vi "Reevaluate Target.vi"(4 "Delay Time (s)":dbl=1.0, 11 "error in (no error)":errorcluster) -> (2 "What to do":string, 3 "error out (no error)":errorcluster)   [LabVIEW 2015]
uses:
  Robot Global Data.vi
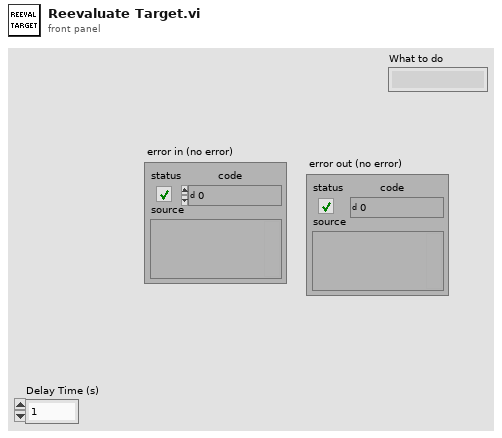
[diagram p1: front panel]
types:
  T1 = cluster{"Goal Left":dbl, "Goal Right":dbl, "Goal Width":dbl}
  T2 = typedef "Relevant Data.ctl" = cluster{"Area":dbl, "CH Area":dbl, "BR Width":dbl, "BR Height":dbl, "BR Left":dbl, "BR Right":dbl}
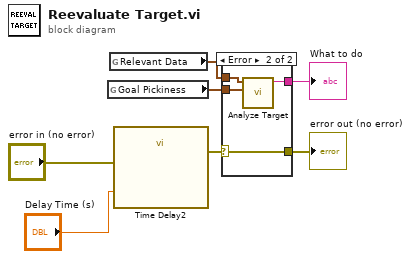
[diagram p0: block diagram]
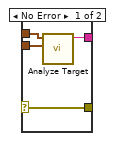
[diagram p2: hidden frame]
diagram:
  n1 = global read "Robot Global Data.vi" "Goal Pickiness"() -> (w3:T1)
  n2 = global read "Robot Global Data.vi" "Relevant Data"() -> (w4:T2[])
  n3 = call "Time Delay2"("error in (no error)"="error in (no error)", "Delay Time (s)"="Delay Time (s)") -> ("error out"=w5:errorcluster)  [unwired: 9 in]
  n4 = case shown="Error" w5 {
    selector: w5 -> [w8 w12]
    tunnel: w4 -> [w11 w15]
    tunnel: w3 -> [w10 w14]
    tunnel: [w9 w13] -> w2
    tunnel: [w8 w12] -> w1
    frame No Error {
      n5 = call "Analyze Target.vi"("Goal Pickiness"=w10, "Relevant Data"=w11) -> ("What to do"=w9:string)  [unwired: 9 in]
    }
    frame Error {
      n6 = call "Analyze Target.vi"("Goal Pickiness"=w14, "Relevant Data"=w15) -> ("What to do"=w13:string)  [unwired: 9 in]
    }
  }
  "What to do" <- w2
  "error out (no error)" <- w1
